vi "Turn ON Results.vi"(8 "ErrorIn":errorcluster, 10 "Command":string, 11 "VISAIn":refnum<visa-resource-name>) -> (0 "ErrorOut":errorcluster, 2 "Data":string, 3 "VISAOut":refnum<visa-resource-name>)   [LabVIEW 2017, in "I28Drivers.lvlib"]
uses:
  I28Drivers.lvlib
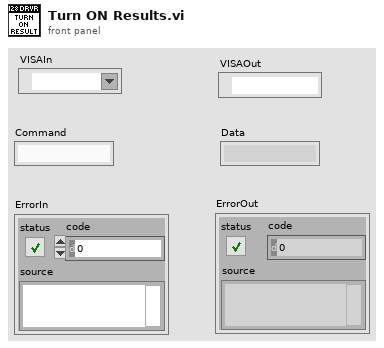
[diagram p1: front panel]
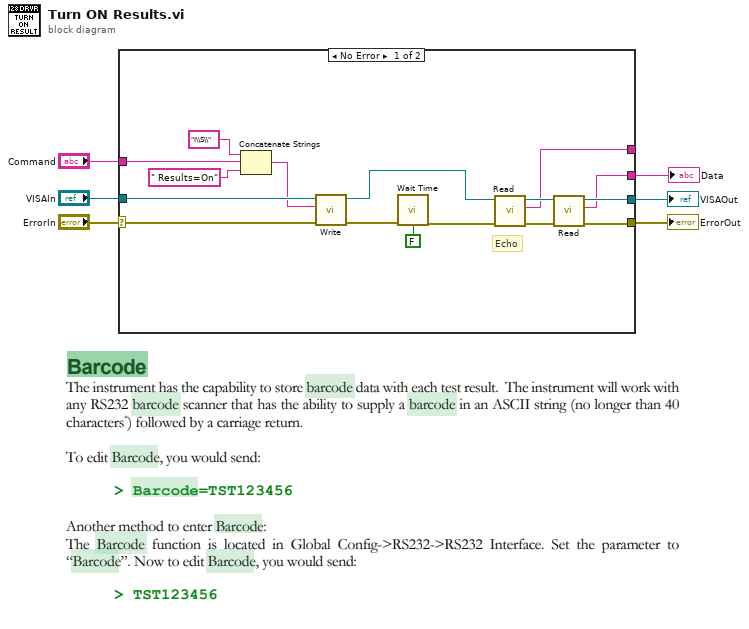
[diagram p0: block diagram]
diagram:
  n1 = case shown="No Error" "ErrorIn" {
    selector: "ErrorIn" -> [w22 w23]
    tunnel: "VISAIn" -> [w21 w24]
    tunnel: "Command" -> [w20 _]
    tunnel: [w15 w23] -> w3
    tunnel: [w13 w24] -> w2
    tunnel: [w12 _] -> w1
    tunnel: [w11 _] -> _
    frame No Error {
      # "Echo"
      n2 = Concatenate Strings("I\\S\\" ("string"), w20, " Results=On" ("string")) -> (w19:string)
      n3 = call "Write.vi"("ErrorIn"=w22, "Command"=w19, "VISAIn"=w21) -> ("ErrorOut"=w9:errorcluster, "VISAOut"=w10:refnum<visa-resource-name>)  [unwired: 7 in]
      n4 = call "Wait Time.vi"("error in"=w9, "Set Time"=FALSE) -> ("error out"=w8:errorcluster)  [unwired: 13 in]
      n5 = call "Read.vi"("ErrorIn"=w8, "VISAIn"=w10) -> ("ErrorOut"=w16:errorcluster, "Data"=w11:string, "VISAOut"=w14:refnum<visa-resource-name>)  [unwired: 7 in]
      n6 = call "Read.vi"("ErrorIn"=w16, "VISAIn"=w14) -> ("ErrorOut"=w15:errorcluster, "Data"=w12:string, "VISAOut"=w13:refnum<visa-resource-name>)  [unwired: 7 in]
    }
    frame Error {
    }
  }
  "ErrorOut" <- w3
  "VISAOut" <- w2
  "Data" <- w1
